vi "Actor Core.vi"(8 "error in":errorcluster, 11 "Universal Card in":refnum<class "Universal Card.lvclass">) -> (0 "error out":errorcluster, 3 "Actor out":refnum<class "Actor.lvclass">)   [LabVIEW 2013, in "Universal Power Meter.lvlib" / "Universal Card.lvclass"]
doc: "(<B>Filename</B>: Actor Framework.lvlib:Actor.lvclass:Actor Core.vi)\n\nReceives messages to the actor, reacts to them, and initiates any error handling that may shut the actor down.\n\nDescendant classes may override this VI to append parallel tasks for the actor to complete while it handles messages. Overrides use the Call Parent Method node."
uses:
  Universal Card.lvclass
  <vilib>/ActorFramework/Actor/Actor.lvclass
  <vilib>/ActorFramework/Message Enqueuer/Message Priority.ctl
  Display Panel/Universal Display/Universal Display.lvclass
  Generic Instrument/Generic Card/Generic Card.lvclass/Generic Card.ctl
  Generic Instrument/Generic Instrument.lvclass
  <vilib>/ActorFramework/Actor/Actor.lvclass/Actor.ctl
  <vilib>/ActorFramework/Message Enqueuer/Message Enqueuer.lvclass/Message Enqueuer.ctl
  Generic Instrument/Generic Card/Generic Card.lvclass
  Display Panel/Abstract Display Messages/Write card number digit Msg/Write card number digit Msg.lvclass/Write card number digit Msg.ctl
  Display Panel/Abstract Display Messages/Measurement Interval number Writer Msg/Measurement Interval number Writer Msg.lvclass/Measurement Interval number Writer Msg.ctl
  Universal Power Meter class/Universal Power Meter.lvclass
  Universal Power Meter Messages/Integrator Start-Stop Msg/Integrator Start-Stop Msg.lvclass/Integrator Start-Stop Msg.ctl
  Display Panel/Abstract Display/Control 1.ctl
  Display Panel/Abstract Display Messages/State Right value from Ref Msg/State Right value from Ref Msg.lvclass/State Right value from Ref Msg.ctl
  Display Panel/Abstract Display Messages/Write time digit Msg/Write time digit Msg.lvclass/Write time digit Msg.ctl
  Display Panel/Universal Display Messages/Updater Msg/Updater Msg.lvclass/Updater Msg.ctl
  Universal Card Messages/WH and AH initialization Msg/WH and AH initialization Msg.lvclass/WH and AH initialization Msg.ctl
  <vilib>/ActorFramework/Message Enqueuer/Init from Existing Queue.vi
  <vilib>/ActorFramework/Message Enqueuer/Enqueue.vi
  <vilib>/ActorFramework/Message Priority Queue/Priority Enqueue.vi
  <vilib>/ActorFramework/Message Enqueuer/Message Enqueuer.lvclass
  Display Panel/Abstract Display Messages/Write card number digit Msg/Write card number digit Msg.lvclass
  Display Panel/Abstract Display Messages/Measurement Interval number Writer Msg/Measurement Interval number Writer Msg.lvclass
  Universal Power Meter Messages/Integrator Start-Stop Msg/Integrator Start-Stop Msg.lvclass
  Display Panel/Abstract Display Messages/State Right value from Ref Msg/State Right value from Ref Msg.lvclass
  Display Panel/Abstract Display Messages/Write time digit Msg/Write time digit Msg.lvclass
  Display Panel/Universal Display Messages/Updater Msg/Updater Msg.lvclass
  Universal Card Messages/WH and AH initialization Msg/WH and AH initialization Msg.lvclass
  Display Panel/Abstract Display/Abstract Display.lvclass
panel:
  out "Val":i32
  out "x <= y?":bool
  out "Array":dbl[](array[numeric])
  out "i":i32
  out "Time has Elapsed":bool
  out "Time":dbl format="%<%H:%M:%S>t"
  out "Start blinking":bool=TRUE
  in  "Stop bit":bool
  out "Warming done":bool
  # "Generic Card Class Core"
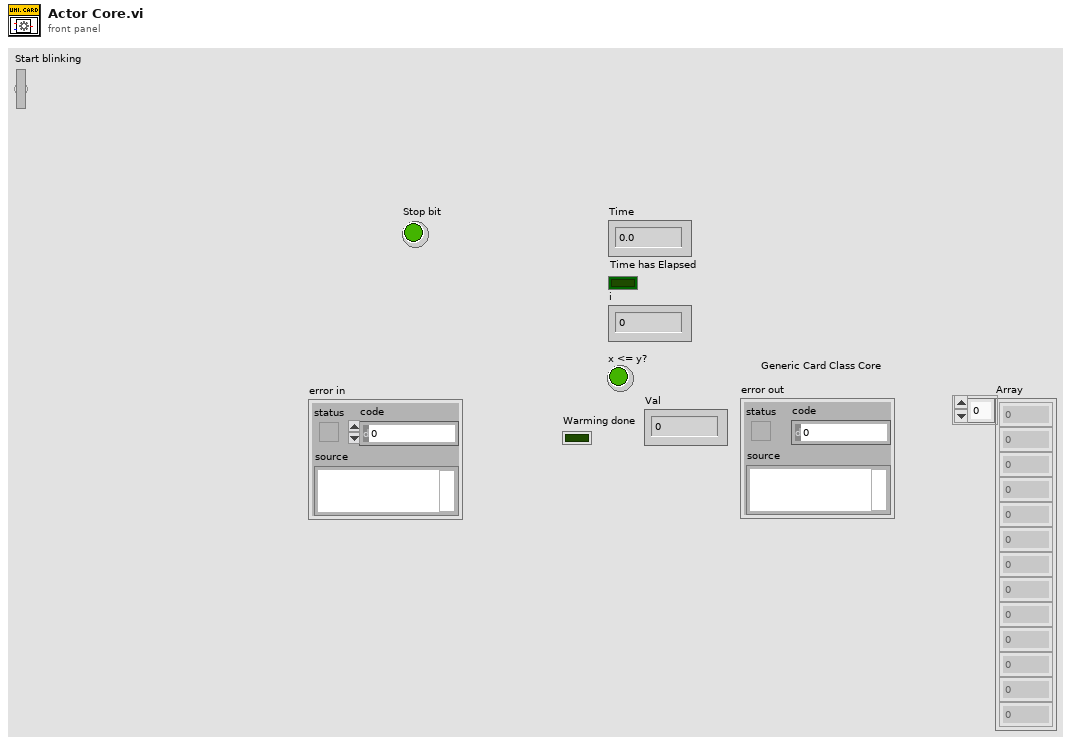
[diagram p1: front panel]
types:
  T1 = typedef "Actor Framework.lvlib/Message Enqueuer.lvclass/Message Priority.ctl" = enum16{"Low", "Normal", "High"}
  T2 = typedef "Display Panel.lvlib/Abstract Display.lvclass/Control 1.ctl" = enum16{"Done", "Warming", "Measuring"}
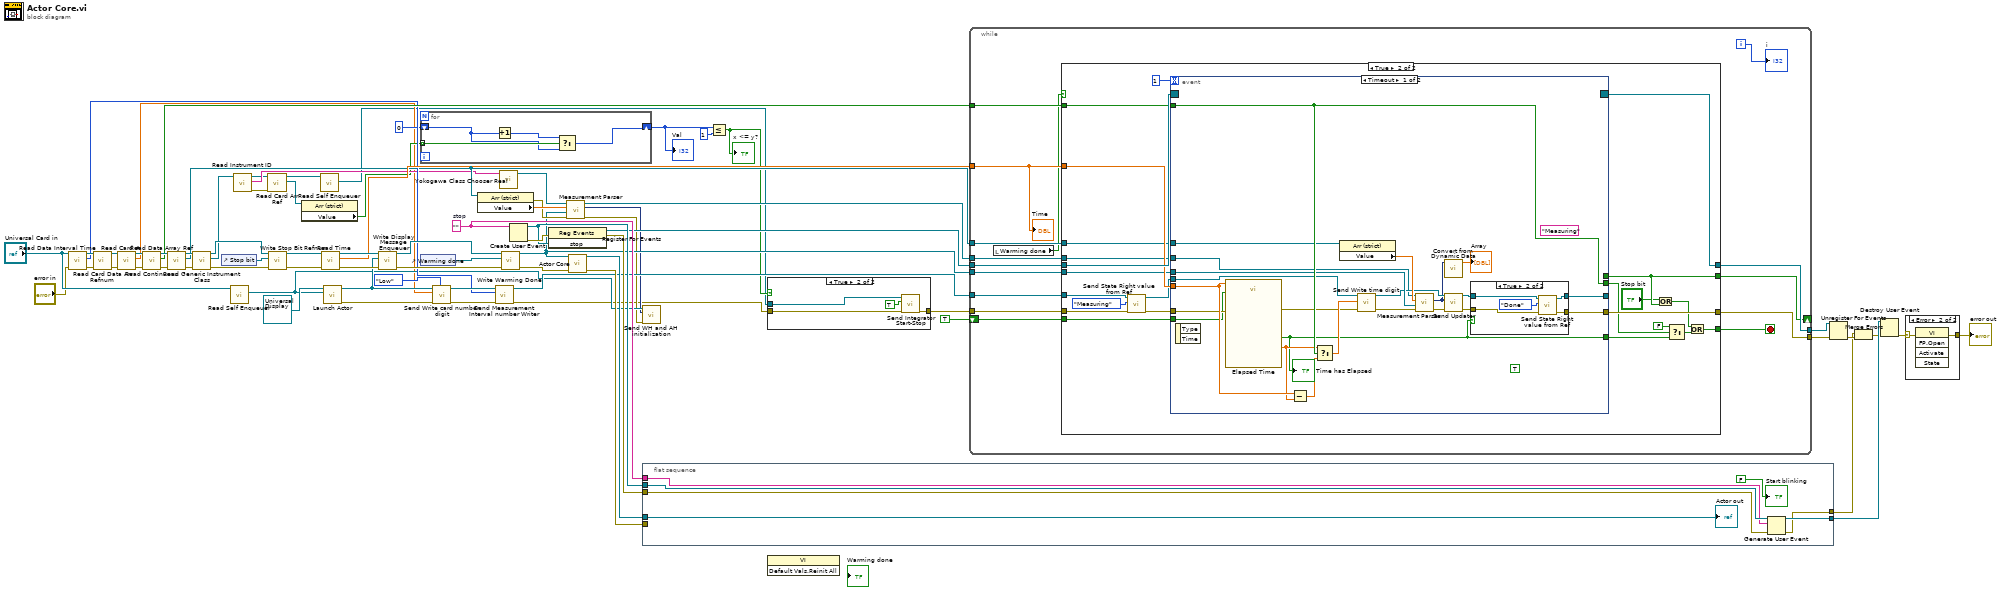
[diagram p0: block diagram]
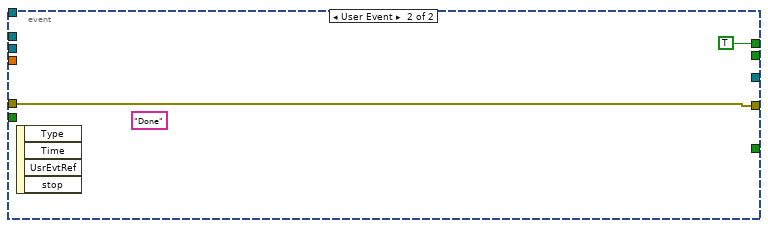
[diagram p6: hidden frame]
diagram:
  w68 = ""  # stop
  n1 = call "Read Data Interval Time.vi"("error in (no error)"="error in", "Generic Card in"="Universal Card in") -> ("error out"=w30:errorcluster, "Data Interval Time"=w29:u16, "Generic Card out"=w32:refnum<class "Universal Card.lvclass">)  [unwired: 7 in]
  n2 = call "Read Card Data Arr  Refnum.vi"("error in (no error)"=w30, "Universal Card in"=w32) -> ("error out"=w64:errorcluster, "Universal Card out"=w65:refnum<class "Universal Card.lvclass">)  [unwired: 7 in, 1 out]
  n3 = call "Read Card #.vi"("error in (no error)"=w64, "Generic Card in"=w65) -> ("error out"=w62:errorcluster, "Card #"=w11:dbl, "Generic Card out"=w63:refnum<class "Universal Card.lvclass">)  [unwired: 7 in]
  n4 = call "Read Continuous.vi"("error in (no error)"=w62, "Generic Card in"=w63) -> ("error out"=w60:errorcluster, "Continuous?"=w48:bool, "Generic Card out"=w61:refnum<class "Universal Card.lvclass">)  [unwired: 7 in]
  n5 = call "Read Data Array Ref.vi"("error in (no error)"=w60, "Generic Card in"=w61) -> ("error out"=w55:errorcluster, "Data Array Ref"=w28:refnum<vi>, "Generic Card out"=w54:refnum<class "Universal Card.lvclass">)  [unwired: 7 in]
  n6 = call "Read Generic Instrument Class.vi"("error in (no error)"=w55, "Generic Card in"=w54) -> ("error out"=w56:errorcluster, "Generic Instrument.lvlib:Generic Instrument.lvclass"=w45:refnum<class "Generic Instrument.lvclass">, "Generic Card out"=w59:refnum<class "Universal Card.lvclass">)  [unwired: 7 in]
  n7 = control-ref of="Stop bit"() -> (w46:refnum<vi>)
  n8 = call <vilib>:"Read Self Enqueuer.vi"("Actor"="Universal Card in") -> ("Self Enqueuer"=w21:refnum<class "Message Enqueuer.lvclass">)  [unwired: 10 in]
  n9 = call-dynamic "Read Instrument ID.vi"("Generic Instrument in"=w45) -> ("error out"=w17:errorcluster, "Instrument ID"=w25:string, "Generic Instrument out"=w18:refnum<class "Generic Instrument.lvclass">)  [unwired: 8 in]
  n10 = call-dynamic "Read Card Arr Ref.vi"("error in (no error)"=w17, "Generic Instrument in"=w18) -> ("Card Arr Ref"=w16:refnum<vi>, "Generic Instrument out"=w9:refnum<class "Generic Instrument.lvclass">)  [unwired: 7 in, 1 out]
  n11 = call "Write Stop Bit Refnum.vi"("error in (no error)"=w56, "Stop Bit Refnum"=w46, "Generic Card in"=w59) -> ("error out"=w57:errorcluster, "Generic Card out"=w58:refnum<class "Universal Card.lvclass">)  [unwired: 7 in]
  n12 = property class="Arr (strict)"(reference=w16) -> ("Value"=w15:bool[])  [unwired: 1 in, 2 out]
  n13 = call <vilib>:"Read Self Enqueuer.vi"("Actor"=w9) -> ("Self Enqueuer"=w8:refnum<class "Message Enqueuer.lvclass">)  [unwired: 10 in]
  n14 = call "Read Time .vi"("error in (no error)"=w57, "Generic Card in"=w58) -> ("error out"=w52:errorcluster, "Time"=w47:dbl, "Generic Card out"=w53:refnum<class "Universal Card.lvclass">)  [unwired: 7 in]
  n15 = call <vilib>:"Launch Actor.vi"("Actor-to-Caller Enqueuer"=w21, "Actor"=refnum<class "Universal Display.lvclass"> refnum ("Display Panel.lvlib:Universal Display.lvclass")) -> ("error out"=w39:errorcluster, "Caller-To-Actor Enqueuer"=w40:refnum<class "Message Enqueuer.lvclass">)  [unwired: 8 in]
  n16 = call "Write Display Message Enqueuer.vi"("error in (no error)"=w52, "Actor Framework.lvlib:Message Enqueuer"=w40, "Generic Card in"=w53) -> ("error out"=w51:errorcluster, "Generic Card out"=w50:refnum<class "Universal Card.lvclass">)  [unwired: 7 in]
  n17 = for {
    tunnel: w15 -> [w77] mode=indexing
    shift-right: [w76] -> w13
    shift-left: 0 -> [w75]
    n18 = Increment(x=w75) -> (x+1=w74:i32)
    n19 = Select(t=w74, s=w77, f=w75) -> (s? t:f=w76:i32)
  }
  "Val" <- w13
  n20 = control-ref of="Warming done"() -> (w71:refnum<vi>)
  n21 = call "Send Write card number digit.vi"("Message Priority (Normal)"=Message_Priority."Low", "error in (no error)"=w39, "Card #"=w11, "Message Enqueuer"=w40) -> ("error out"=w36:errorcluster, "Message Enqueuer out"=w35:refnum<class "Message Enqueuer.lvclass">)  [unwired: 6 in]
  n22 = property class="Arr (strict)"(reference=w28) -> (error out=w26:errorcluster, "Value"=w27:dbl[])  [unwired: 1 in, 1 out]
  n23 = call "Send Measurement Interval number Writer.vi"("error in (no error)"=w36, "Update Time"=w29, "Message Enqueuer"=w35) -> ("error out"=w7:errorcluster, "Message Enqueuer out"=w34:refnum<class "Message Enqueuer.lvclass">)  [unwired: 7 in]
  n24 = call "Yokogawa Class Chooser Real.vi"("Incoming ID in"=w25) -> ("Universal Power Meter out"=w24:refnum<class "Universal Power Meter.lvclass">)  [unwired: 9 in, 1 out]
  n25 = call "Write Warming Done.vi"("error in (no error)"=w51, "Warming Done"=w71, "Generic Card in"=w50) -> ("error out"=w66:errorcluster, "Generic Card out"=w22:refnum<class "Universal Card.lvclass">)  [unwired: 7 in]
  n26 = Create User Event(user event datatype=w68) -> (user event=w69:refnum<user-event>, error out=w70:errorcluster)  [unwired: 1 in]
  n27 = register-events(error in=w70, w69) -> (reference out=w49:refnum<event-registration>, error out=w67:errorcluster)  [unwired: 1 in]
  n28 = call-dynamic "Measurement Parser.vi"("error in (no error)"=w26, "Universal Power Meter.lvlib:Universal Card.lvclass"=w22, "Data Array"=w27, "Universal Power Meter in"=w24) -> ("error out"=w19:errorcluster, "Waveform Graph"=w20:dynamicdata, "Universal Power Meter out"=w23:refnum<class "Universal Power Meter.lvclass">)  [unwired: 5 in]
  n29 = call-parent "Actor Core.vi"("error in"=w66, "Generic Card in"=w22) -> ("error out"=w73:errorcluster, "Actor out"=w72:refnum<class "Actor.lvclass">)  [unwired: 8 in]
  n30 = call "Send WH and AH initialization.vi"("error in (no error)"=w19, "Dynamic Data"=w20, "Message Enqueuer"=w21) -> ()  [unwired: 7 in, 2 out]
  n31 = flat-sequence {
    tunnel: w73 -> [_]
    tunnel: w72 -> [w80]
    tunnel: w69 -> [w84]
    tunnel: w68 -> [w83]
    tunnel: w67 -> [w82]
    tunnel: [w79] -> w43
    tunnel: [w78] -> w3
    frame #0 {
      n32 = Generate User Event(user event=w84, event data cluster=w83, error in=w82) -> (user event out=w79:refnum<user-event>, error out=w78:errorcluster)  [unwired: 1 in]
      "Start blinking" <- FALSE ("stop blinking")
      "Actor out" <- w80
    }
  }
  n33 = Less Or Equal?(x=w13, y=1) -> (x <= y?=w10:bool)
  "x <= y?" <- w10
  n34 = case shown="True" w10 {
    tunnel: w8 -> [_ w88]
    tunnel: w7 -> [w85 w87]
    tunnel: [w85 w86] -> w6
    frame False {
    }
    frame True {
      n35 = call "Send Integrator Start-Stop.vi"("error in (no error)"=w87, "Start/Stop (F: Stop)"=TRUE, "Message Enqueuer"=w88) -> ("error out"=w86:errorcluster)  [unwired: 7 in, 1 out]
    }
  }
  n36 = invoke class="VI" method="Default Vals.Reinit All"() -> ()  [unwired: 3 in, 3 out]
  n37 = while {
    tunnel: w49 -> [w104]
    tunnel: [w103] -> w42
    tunnel: w48 -> [w102]
    tunnel: w47 -> [w101]
    tunnel: w34 -> [w100]
    tunnel: w6 -> [w99]
    tunnel: [w98] -> w41
    tunnel: w28 -> [w97]
    tunnel: w22 -> [w96]
    shift-right: [w93] -> _
    shift-left: TRUE -> [w95]
    tunnel: w23 -> [w91]
    i -> [w94]
    stop <- w92 stop-if-true
    n38 = local read "Warming done"() -> (w90:bool)
    n39 = case shown="True" w90 {
      tunnel: w104 -> [w105 w130]
      tunnel: [w105 w129] -> w103
      tunnel: w102 -> [_ w128]
      tunnel: w101 -> [_ w127]
      tunnel: w100 -> [_ w126]
      tunnel: w99 -> [w107 w125]
      tunnel: [w107 w124] -> w98
      tunnel: w97 -> [_ w123]
      tunnel: w96 -> [_ w122]
      tunnel: w95 -> [w106 w121]
      tunnel: [w106 w120] -> w93
      tunnel: [_ w119] -> w92
      tunnel: w91 -> [_ w118]
      frame False {
      }
      frame True {
        n40 = call "Send State Right value from Ref.vi"("error in (no error)"=w125, "States"=Control_1."Measuring", "Message Enqueuer"=w126) -> ("error out"=w109:errorcluster, "Message Enqueuer out"=w110:refnum<class "Message Enqueuer.lvclass">)  [unwired: 7 in]
        n41 = event shown="[0] Timeout" {
          selector: w130 -> [_ _]
          dyn-events: [_ _] -> w129
          timeout: 1 -> [_ _]
          tunnel: [_ TRUE ("Stop Button")] -> w120
          tunnel: w128 -> [w153 _]
          tunnel: [w153 _] -> w115
          tunnel: w127 -> [w152 _]
          tunnel: [w141 _] -> w111
          tunnel: w110 -> [w150 _]
          tunnel: w109 -> [w147 w161]
          tunnel: [w140 _] -> _
          tunnel: [w139 w161] -> w124
          tunnel: w123 -> [w145 _]
          tunnel: w122 -> [w143 _]
          tunnel: w121 -> [w142 _]
          tunnel: w118 -> [w131 _]
          event Timeout {
            (unwired) TRUE ("Blink? Ref")
            (unwired) "Measuring" ("Caption")
            n42 = event-data() -> ()  [unwired: 1 in, 2 out]
            n43 = call "Elapsed Time"("Time Target (s)"=w152, "Reset"=w142, "error in (no error)"=w147) -> ("Elapsed Time (s)"=w148:dbl, "Time has Elapsed"=w141:bool, "error out"=w146:errorcluster)  [unwired: 9 in, 5 out]
            "Time has Elapsed" <- w141
            n44 = Subtract(x=w152, y=w148) -> (x-y=w151:dbl)
            n45 = Select(t=w148, s=w153, f=w151) -> (s? t:f=w149:dbl)
            n46 = property class="Arr (strict)"(reference=w145) -> ("Value"=w144:dbl[])  [unwired: 1 in, 2 out]
            n47 = call "Send Write time digit.vi"("error in (no error)"=w146, "Time"=w149, "Message Enqueuer"=w150) -> ("error out"=w133:errorcluster, "Message Enqueuer out"=w138:refnum<class "Message Enqueuer.lvclass">)  [unwired: 7 in]
            n48 = call-dynamic "Measurement Parser.vi"("error in (no error)"=w133, "Universal Power Meter.lvlib:Universal Card.lvclass"=w143, "Data Array"=w144, "Universal Power Meter in"=w131) -> ("error out"=w132:errorcluster, "Waveform Graph"=w134:dynamicdata)  [unwired: 5 in, 1 out]
            n49 = call "Convert from Dynamic Data"("Dynamic Data Type"=w134) -> ("Array"=→"Array":dbl[])  [unwired: 3 in]
            n50 = call "Send Updater.vi"("error in (no error)"=w132, "Waveform Chart"=w134, "Message Enqueuer"=w138) -> ("error out"=w136:errorcluster, "Message Enqueuer out"=w137:refnum<class "Message Enqueuer.lvclass">)  [unwired: 7 in]
            n51 = case shown="True" w141 {
              tunnel: w137 -> [w155 w160]
              tunnel: [w155 w159] -> w140
              tunnel: w136 -> [w154 w158]
              tunnel: [w154 w157] -> w139
              frame False {
              }
              frame True {
                n52 = call "Send State Right value from Ref.vi"("error in (no error)"=w158, "States"=Control_1."Done", "Message Enqueuer"=w160) -> ("error out"=w157:errorcluster, "Message Enqueuer out"=w159:refnum<class "Message Enqueuer.lvclass">)  [unwired: 7 in]
              }
            }
          }
          event User Event {
            (unwired) "Done" ("Caption")
            n53 = event-data() -> ()  [unwired: 1 in, 4 out]
          }
        }
        n54 = Or(x="Stop bit", y=w120) -> (x .or. y?=w113:bool)
        n55 = Select(t=FALSE ("f"), s=w115, f=w111) -> (s? t:f=w112:bool)
        n56 = Or(x=w113, y=w112) -> (x .or. y?=w119:bool)
      }
    }
    "Time" <- w101
    "i" <- w94
  }
  n57 = Unregister For Events(event registration refnum=w42, error in=w41) -> (error out=w5:errorcluster)
  n58 = Merge Errors(w3, w5) -> (w2:errorcluster)
  n59 = Destroy User Event(user event=w43, error in=w2) -> (error out=w1:errorcluster)
  n60 = case shown="Error" w1 {
    selector: w1 -> [w163 w165]
    tunnel: [w163 w164] -> w4
    frame No Error {
    }
    frame Error {
      n61 = invoke class="VI" method="FP.Open"(error in=w165) -> (error out=w164:errorcluster)  [unwired: 4 in, 4 out]
    }
  }
  "error out" <- w4
